vi "FPGA uint limit counter with reset.vi"(1 "dt":u32, 2 "Reset":bool, 3 "Limit":u32) -> (0 "Overflow":bool)   [LabVIEW 2010]
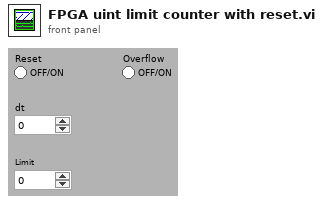
[diagram p1: front panel]
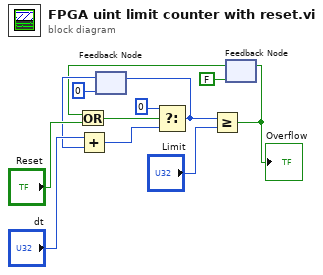
[diagram p0: block diagram]
diagram:
  n1 = feedback #1(u32 0 ("t")) -> (w5:u32)
  n2 = Add(x="dt", y=w5) -> (x+y=w7:u32)
  n3 = feedback #2(FALSE) -> (w3:bool)
  n4 = Or(x=w3, y="Reset") -> (x .or. y?=w4:bool)
  n5 = Select(t=u32 0, s=w4, f=w7) -> (s? t:f=w11:u32)
  n6 = feedback-in #1(w11) -> ()
  n7 = Greater Or Equal?(x=w11, y="Limit") -> (x >= y?=w2:bool)
  "Overflow" <- w2
  n8 = feedback-in #2(w2) -> ()
